vi "Get Default Log File Path.vi"(8 "error in":errorcluster, 10 "Target Type":T1(ring)) -> (0 "error out":errorcluster, 2 "Log File Path String Array":string[](array[string]))   [LabVIEW 2019, in "Telemetry System Explorer.lvlib"]
uses:
  Telemetry System Explorer.lvlib
  <vilib>/NI VeriStand/Custom Device Tools/Custom Device Utility Library/Custom Device Utility Library.lvlib
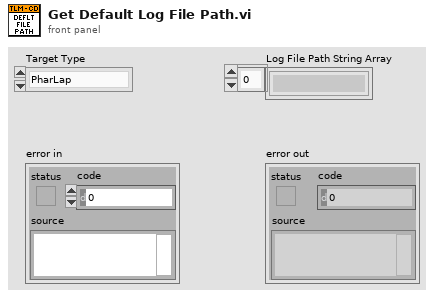
[diagram p1: front panel]
types:
  T1 = enum16{"PharLap", "VxWorks", "Windows", "Linux_32_ARM", "Linux_x64"}
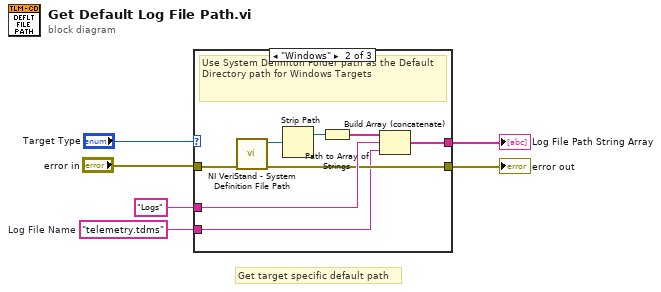
[diagram p0: block diagram]
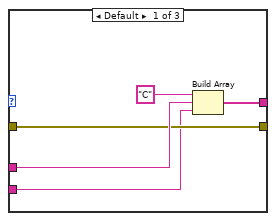
[diagram p2: hidden frame]
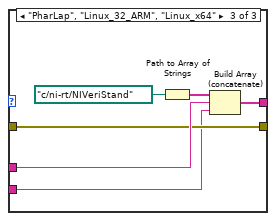
[diagram p3: hidden frame]
diagram:
  w1 = "telemetry.tdms"  # Log File Name
  # "Get target specific default path"
  n1 = case shown="\"Windows\"" "Target Type" {
    tunnel: [w10 w18 w24] -> w6
    tunnel: "Logs" -> [w11 w19 w25]
    tunnel: "error in" -> [w9 w17 w22]
    tunnel: [w9 w16 w22] -> w3
    tunnel: w1 -> [w7 w12 w20]
    frame Default {
      n2 = Build Array("C" ("element"), w11, w7) -> (w10:string[])
    }
    frame "Windows" {
      # "Use System Definiton Folder path as the Default Directory path for Windows Targets"
      n3 = call <vilib>:"NI VeriStand - System Definition File Path.vi"("error in (no error)"=w17) -> ("error out"=w16:errorcluster, "SDF path"=w15:path)  [unwired: 9 in]
      n4 = Strip Path(path=w15) -> (stripped path=w14:path)  [unwired: 1 out]
      n5 = Path to Array of Strings(0:w14) -> (2:w13:string[])  [unwired: 1 out]
      n6 = Build Array (concatenate)(w13, w19, w12) -> (w18:string[])
    }
    frame "PharLap", "Linux_32_ARM", "Linux_x64" {
      n7 = Path to Array of Strings(0:path "c:/ni-rt/NIVeriStand" ("path")) -> (2:w21:string[])  [unwired: 1 out]
      n8 = Build Array (concatenate)(w21, w25, w20) -> (w24:string[])
    }
  }
  "Log File Path String Array" <- w6
  "error out" <- w3
